vi "Track Graph with Mouse.vi"(10 "Y":dbl, 11 "WaveformGraph in":refnum<vi>) -> ()   [LabVIEW 2013, in "main.lvlib"]
uses:
  main.lvlib
  USER32.DLL
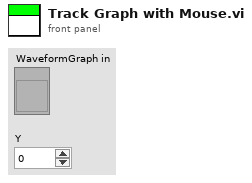
[diagram p1: front panel]
types:
  T1 = typedef "LVRectTypeDef.ctl" = cluster{"Left":i16, "Top":i16, "Right":i16, "Bottom":i16}
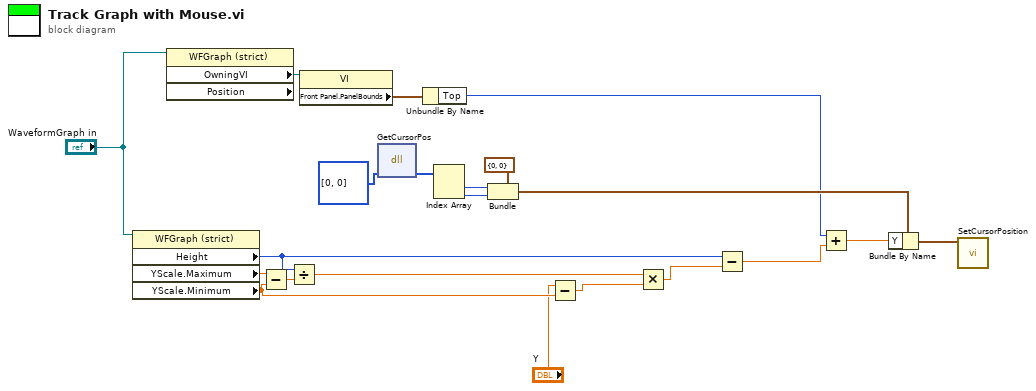
[diagram p0: block diagram]
diagram:
  n1 = property class="WFGraph (strict)"(reference="WaveformGraph in") -> ("Height"=w16:u32, "YScale.Maximum"=w3:dbl, "YScale.Minimum"=w14:dbl)  [unwired: 1 in, 2 out]
  n2 = property class="WFGraph (strict)" props=["OwningVI", "Position"](reference="WaveformGraph in") -> ("OwningVI"=w7:refnum<vi>)  [unwired: 1 in, 3 out]
  n3 = Subtract(x=w3, y=w14) -> (x-y=w4:dbl)
  n4 = Divide(x=w16, y=w4) -> (x/y=w5:dbl)
  n5 = property class="VI"(reference=w7) -> ("Front Panel.PanelBounds"=w8:T1)  [unwired: 1 in, 2 out]
  n6 = dll-call lib="USER32.DLL" fn="GetCursorPos"("Position"=i32[] [0, 0]) -> ("Position"=w2:i32[])  [unwired: 4 in, 2 out]
  n7 = Unbundle By Name(w8) -> ("Top"=w12:i16)
  n8 = Index Array(array=w2) -> (element #1=w9:i32, element #2=w10:i32)  [unwired: 2 in]
  n9 = Bundle(cluster=cluster{"X":i32, "Y":i32} {"X"=0, "Y"=0}, "X"=w9, "Y"=w10) -> (w19:cluster{"X":i32, "Y":i32})
  n10 = Subtract(x="Y", y=w14) -> (x-y=w15:dbl)
  n11 = Multiply(x=w5, y=w15) -> (x*y=w17:dbl)
  n12 = Subtract(x=w16, y=w17) -> (x-y=w18:dbl)
  n13 = Add(x=w12, y=w18) -> (x+y=w20:dbl)
  n14 = Bundle By Name(cluster=w19, "Y"=w20) -> (w21:cluster{"X":i32, "Y":i32})
  n15 = call "SetCursorPosition.vi"("XY"=w21) -> ()  [unwired: 11 in]
